vi "save channels to separate tiff series.vi"(8 "frame number in":i32, 9 "last frame":bool, 11 "image data in":dbl[][](array[numeric])) -> ()   [LabVIEW 2012]
uses:
  Custom Controls/file format type def.ctl
  GFG/GFGpathGet.vi
  GFG/GFGnumericGet.vi
  GFG/GFG library.lvlib
  Libtiff3/libtiff3.llb/libtiff3.lvlib
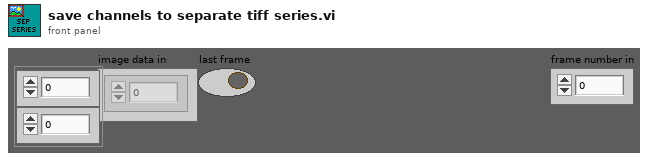
[diagram p1: front panel]
types:
  T1 = typedef "file format type def.ctl" = enum16{"16bit raw", "32bit raw", "16bit multi-tiff (interleave)", "16bit multi-tiff (separate)", "16bit multi-tiff (stacked)", "32bit multi-tiff (interleave)", "32bit multi-tiff (separate)", "32bit multi-tiff (stacked)", "16bit tiff series (interleave)", "16bit tiff series (separate)", "16bit tiff series (stacked)", "32bit tiff series (interleave)", "32bit tiff series (separate)", "32bit tiff series (stacked)"}
  T2 = cluster{"no..of.frames.to.acquire":dbl, "x.pixels":dbl, "y.pixels":dbl, "x.pixel.sz":dbl, "y.pixel.sz":dbl}
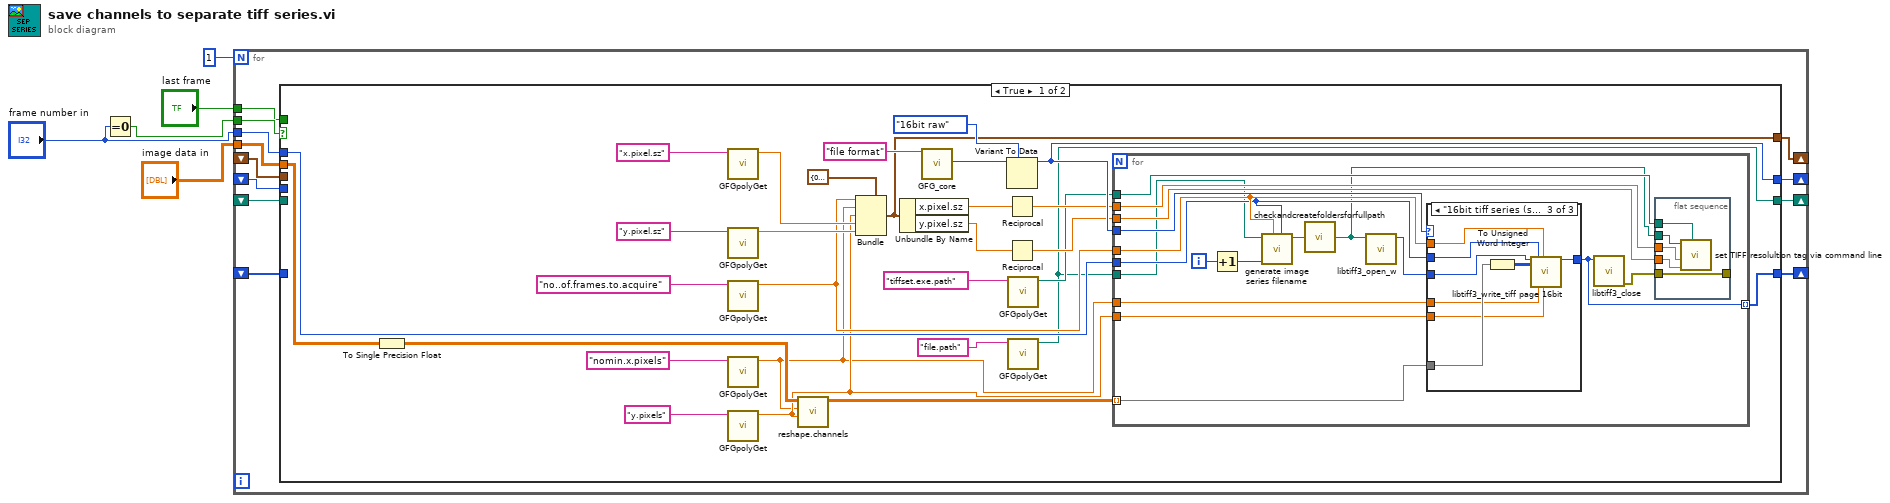
[diagram p0: block diagram]
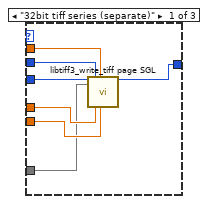
[diagram p2: hidden frame]
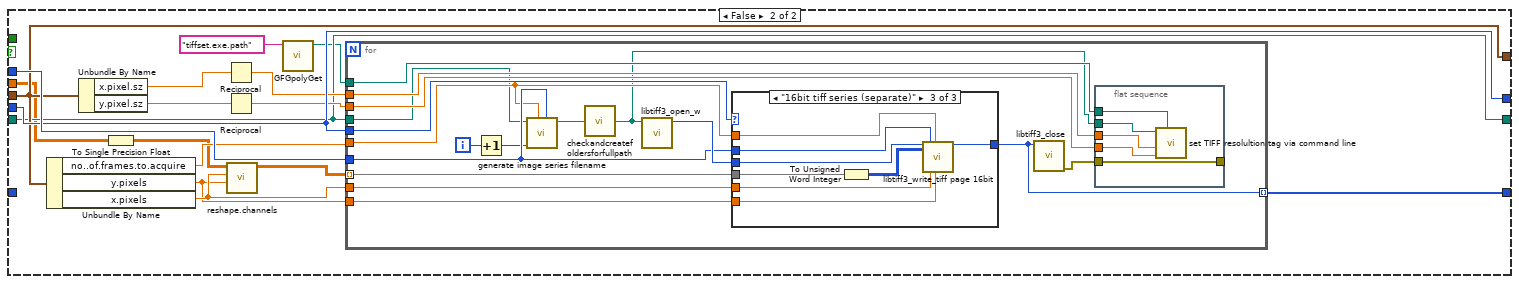
[diagram p4: hidden frame]
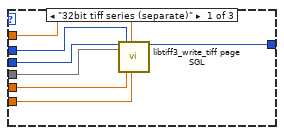
[diagram p5: hidden frame]
diagram:
  n1 = Equal To 0?(x="frame number in") -> (x = 0?=w4:bool)
  n2 = for {
    N: 1 -> [_]
    tunnel: w4 -> [w17]
    shift-right: [w16] -> _
    shift-left: _ -> [w15]
    tunnel: "image data in" -> [w14]
    shift-right: [w13] -> _
    shift-left: _ -> [w12]
    shift-right: [w11] -> _
    shift-left: _ -> [w10]
    shift-right: [w9] -> _
    shift-left: _ -> [w8]
    tunnel: "last frame" -> [w7]
    tunnel: "frame number in" -> [w6]
    n3 = case shown="True" w17 {
      tunnel: w12 -> [_ w99]
      tunnel: [w31 w97] -> w16
      tunnel: w15 -> [_ _]
      tunnel: w14 -> [w21 w88]
      tunnel: [w34 w99] -> w13
      tunnel: [w30 w98] -> w11
      tunnel: w10 -> [_ w98]
      tunnel: [w23 w91] -> w9
      tunnel: w8 -> [_ w91]
      tunnel: w7 -> [_ _]
      tunnel: w6 -> [w32 w101]
      frame True {
        n4 = To Single Precision Float(number=w21) -> (single precision float=w22:sgl[][])
        n5 = call-poly "GFGpolyGet.vi"("Variable Name in"="x.pixel.sz" ("Tag in")) -> ("Numeric"=w37:dbl)  [unwired: 9 in, 1 out]
        n6 = call-poly "GFGpolyGet.vi"("Variable Name in"="y.pixel.sz" ("Tag in")) -> ("Numeric"=w36:dbl)  [unwired: 9 in, 1 out]
        n7 = call-poly "GFGpolyGet.vi"("Variable Name in"="no..of.frames.to.acquire") -> ("Numeric"=w33:dbl)  [unwired: 9 in, 1 out]
        n8 = call-poly "GFGpolyGet.vi"("Variable Name in"="nomin.x.pixels" ("Tag in")) -> ("Numeric"=w18:dbl)  [unwired: 9 in, 1 out]
        n9 = call-poly "GFGpolyGet.vi"("Variable Name in"="y.pixels" ("Tag in")) -> ("Numeric"=w19:dbl)  [unwired: 9 in, 1 out]
        n10 = call "reshape.channels.vi"("y.pixels"=w19, "x.pixels"=w18, "element"=w22) -> ("Array"=w20:dbl[][][])  [unwired: 8 in]
        n11 = Bundle(cluster=T2 {"no..of.frames.to.acquire"=0.0, "x.pixels"=0.0, "y.pixels"=0.0, "x.pixel.sz"=0.0, "y.pixel.sz"=0.0} ("output cluster"), "no..of.frames.to.acquire"=w33, "x.pixels"=w18, "y.pixels"=w19, "x.pixel.sz"=w37, "y.pixel.sz"=w36) -> (w30:T2)
        n12 = Unbundle By Name(w30) -> ("x.pixel.sz"=w26:dbl, "y.pixel.sz"=w27:dbl)
        n13 = call "GFG_core.vi"("Variable Name in"="file format") -> ("Variant Out"=w45:variant)  [unwired: 12 in, 6 out]
        n14 = Variant To Data(type=file_format_type_def."16bit raw" ("file format"), Variant=w45) -> (data=w34:T1)  [unwired: 1 in, 1 out]
        n15 = Reciprocal(x=w26) -> (1/x=w28:dbl)
        n16 = Reciprocal(x=w27) -> (1/x=w29:dbl)
        n17 = call-poly "GFGpolyGet.vi"("Variable Name in"="tiffset.exe.path") -> ("Path"=w24:path)  [unwired: 9 in, 1 out]
        n18 = call-poly "GFGpolyGet.vi"("Variable Name in"="file.path") -> ("Path"=w23:path)  [unwired: 9 in, 1 out]
        n19 = for {
          tunnel: w34 -> [w63]
          tunnel: w18 -> [w61]
          tunnel: w19 -> [w60]
          tunnel: w33 -> [w58]
          tunnel: w32 -> [w57]
          tunnel: [w56] -> w31 mode=indexing
          tunnel: w29 -> [w54]
          tunnel: w28 -> [w53]
          tunnel: w24 -> [w52]
          tunnel: w23 -> [w51]
          tunnel: w20 -> [w48] mode=indexing
          i -> [w50]
          n20 = Increment(x=w50) -> (x+1=w49:i32)
          n21 = call "generate image series filename.vi"("frame number in"=w57, "no..of.frames.to.acquire"=w58, "channel"=w49, "Path IN"=w51) -> ("appended path"=w59:path)  [unwired: 7 in]
          n22 = call "checkandcreatefoldersforfullpath.vi"("Path IN"=w59) -> ("Path OUT"=w47:path)  [unwired: 4 in]
          n23 = call "libtiff3_open_w.vi"("Input path"=w47) -> ("handle"=w62:i32)  [unwired: 9 in, 1 out]
          n24 = case shown="\"16bit tiff series (separate)\"" w63 {
            tunnel: w48 -> [w69 _ w81]
            tunnel: w62 -> [w72 w76 w82]
            tunnel: w57 -> [w73 _ w83]
            tunnel: w58 -> [w74 _ w84]
            tunnel: [w75 w76 w77] -> w56
            tunnel: w61 -> [w70 _ w79]
            tunnel: w60 -> [w71 _ w78]
            frame "32bit tiff series (separate)" {
              n25 = call "libtiff3_write_tiff page SGL.vi"("Handle"=w72, "Image Pixels (Float)"=w69, "page"=w73, "x.pixels"=w70, "totalpages"=w74, "y.pixels"=w71) -> ("Handle out"=w75:i32)  [unwired: 12 in, 1 out]
            }
            frame Default {
            }
            frame "16bit tiff series (separate)" {
              n26 = To Unsigned Word Integer(number=w81) -> (unsigned 16bit integer=w80:u16[][])
              n27 = call "libtiff3_write_tiff page 16bit.vi"("Handle"=w82, "Image Pixels (U16)"=w80, "page"=w83, "x.pixels"=w79, "totalpages"=w84, "y.pixels"=w78) -> ("Handle out"=w77:i32)  [unwired: 12 in, 1 out]
            }
          }
          n28 = call "libtiff3_close.vi"("Handle"=w56) -> ("error out"=w55:errorcluster)  [unwired: 9 in]
          n29 = flat-sequence {
            tunnel: w55 -> [w66]
            tunnel: w53 -> [w68]
            tunnel: w54 -> [w67]
            tunnel: [w66] -> _
            tunnel: w52 -> [w65]
            tunnel: w47 -> [w64]
            frame #0 {
              n30 = call "set TIFF resolultion tag via command line.vi"("tiffset.exe file path"=w65, "y pixels per m"=w67, "x pixels per m"=w68, "TIFF file path"=w64) -> ()  [unwired: 8 in]
            }
          }
        }
      }
      frame False {
        n31 = Unbundle By Name(w98) -> ("no..of.frames.to.acquire"=w100:dbl, "y.pixels"=w89:dbl, "x.pixels"=w90:dbl)
        n32 = Unbundle By Name(w98) -> ("x.pixel.sz"=w93:dbl, "y.pixel.sz"=w94:dbl)
        n33 = To Single Precision Float(number=w88) -> (single precision float=w87:sgl[][])
        n34 = Reciprocal(x=w93) -> (1/x=w95:dbl)
        n35 = Reciprocal(x=w94) -> (1/x=w96:dbl)
        n36 = call "reshape.channels.vi"("y.pixels"=w89, "x.pixels"=w90, "element"=w87) -> ("Array"=w86:dbl[][][])  [unwired: 8 in]
        n37 = call-poly "GFGpolyGet.vi"("Variable Name in"="tiffset.exe.path") -> ("Path"=w85:path)  [unwired: 9 in, 1 out]
        n38 = for {
          tunnel: w101 -> [w116]
          tunnel: w100 -> [w115]
          tunnel: w99 -> [w114]
          tunnel: w89 -> [w113]
          tunnel: w90 -> [w112]
          tunnel: [w111] -> w97 mode=indexing
          tunnel: w96 -> [w109]
          tunnel: w95 -> [w108]
          tunnel: w91 -> [w107]
          tunnel: w86 -> [w106] mode=indexing
          tunnel: w85 -> [w105]
          i -> [w104]
          n39 = Increment(x=w104) -> (x+1=w103:i32)
          n40 = call "generate image series filename.vi"("frame number in"=w116, "no..of.frames.to.acquire"=w115, "channel"=w103, "Path IN"=w107) -> ("appended path"=w117:path)  [unwired: 7 in]
          n41 = call "checkandcreatefoldersforfullpath.vi"("Path IN"=w117) -> ("Path OUT"=w102:path)  [unwired: 4 in]
          n42 = call "libtiff3_open_w.vi"("Input path"=w102) -> ("handle"=w118:i32)  [unwired: 9 in, 1 out]
          n43 = case shown="\"16bit tiff series (separate)\"" w114 {
            tunnel: w106 -> [w124 _ w136]
            tunnel: w118 -> [w127 w131 w137]
            tunnel: w116 -> [w128 _ w138]
            tunnel: w115 -> [w129 _ w139]
            tunnel: [w130 w131 w132] -> w111
            tunnel: w112 -> [w125 _ w134]
            tunnel: w113 -> [w126 _ w133]
            frame "32bit tiff series (separate)" {
              n44 = call "libtiff3_write_tiff page SGL.vi"("Handle"=w127, "Image Pixels (Float)"=w124, "page"=w128, "x.pixels"=w125, "totalpages"=w129, "y.pixels"=w126) -> ("Handle out"=w130:i32)  [unwired: 12 in, 1 out]
            }
            frame Default {
            }
            frame "16bit tiff series (separate)" {
              n45 = To Unsigned Word Integer(number=w136) -> (unsigned 16bit integer=w135:u16[][])
              n46 = call "libtiff3_write_tiff page 16bit.vi"("Handle"=w137, "Image Pixels (U16)"=w135, "page"=w138, "x.pixels"=w134, "totalpages"=w139, "y.pixels"=w133) -> ("Handle out"=w132:i32)  [unwired: 12 in, 1 out]
            }
          }
          n47 = call "libtiff3_close.vi"("Handle"=w111) -> ("error out"=w110:errorcluster)  [unwired: 9 in]
          n48 = flat-sequence {
            tunnel: w110 -> [w121]
            tunnel: w108 -> [w123]
            tunnel: w109 -> [w122]
            tunnel: [w121] -> _
            tunnel: w105 -> [w120]
            tunnel: w102 -> [w119]
            frame #0 {
              n49 = call "set TIFF resolultion tag via command line.vi"("tiffset.exe file path"=w120, "y pixels per m"=w122, "x pixels per m"=w123, "TIFF file path"=w119) -> ()  [unwired: 8 in]
            }
          }
        }
      }
    }
  }
